vi "CleanUp.vi"(8 "error in (no error)":errorcluster, 11 "TestTestResult in":refnum<class "_TextTestResult.lvclass">) -> (0 "error out":errorcluster, 3 "TestTestResult out":refnum<class "_TextTestResult.lvclass">)   [LabVIEW 2013, in "_TextTestResult.lvclass"]
uses:
  _TextTestResult.lvclass
  TestResult/TestResult.lvclass
panel:
  # "JKI VI Tester for LabVIEW\nhttp://jkisoft.com/vi-tester\nCopyright (C) 2007-2009, JKI <info@jkisoft.com>\nALL RIGHTS RESERVED"
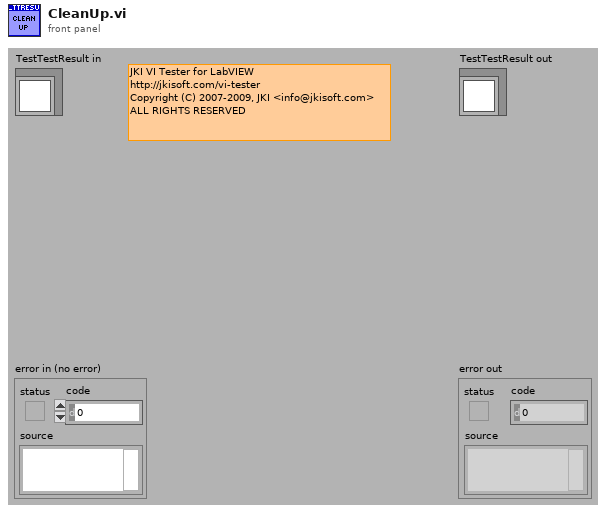
[diagram p1: front panel]
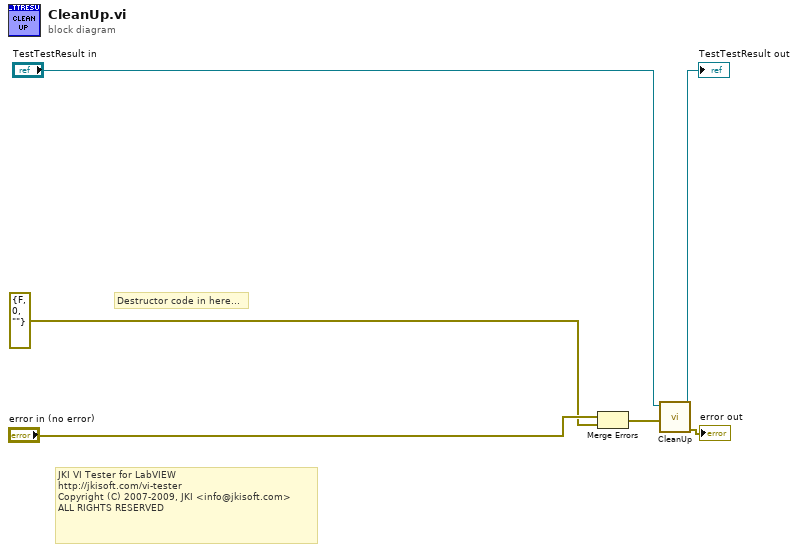
[diagram p0: block diagram]
diagram:
  # "JKI VI Tester for LabVIEW\nhttp://jkisoft.com/vi-tester\nCopyright (C) 2007-2009, JKI <info@jkisoft.com>\nALL RIGHTS RESERVED"
  # "Destructor code in here..."
  n1 = Merge Errors("error in (no error)", errorcluster {"status"=FALSE, "code"=0, "source"=""} ("error in (no error)")) -> (w3:errorcluster)
  n2 = call-parent "CleanUp.vi"("error in (no error)"=w3, "TestResult in"="TestTestResult in") -> ("error out"=→"error out":errorcluster, "TestResult out"=→"TestTestResult out":refnum<class "_TextTestResult.lvclass">)  [unwired: 8 in]
